vi "log SET errors.vi"(8 "error in (no error)":errorcluster, 11 "Channel in":refnum<class "Channel.lvclass">) -> (0 "error out":errorcluster, 3 "Channel out":refnum<class "Channel.lvclass">)   [LabVIEW 2018, in "Channel.lvclass"]
uses:
  Channel.lvclass
  Channel.lvclass/Channel.ctl
  Sim_Ixon_Ultra/Sim_Ixon_Ultra.lvclass
  C:/Users/Denis/Desktop/S4ACS/S4ACS/Simulated_CCD_Camera/Simulated Camera.lvclass
  Simulated_CCD_Camera/Simulated Camera.lvclass
panel:
  out "SET errors":T1
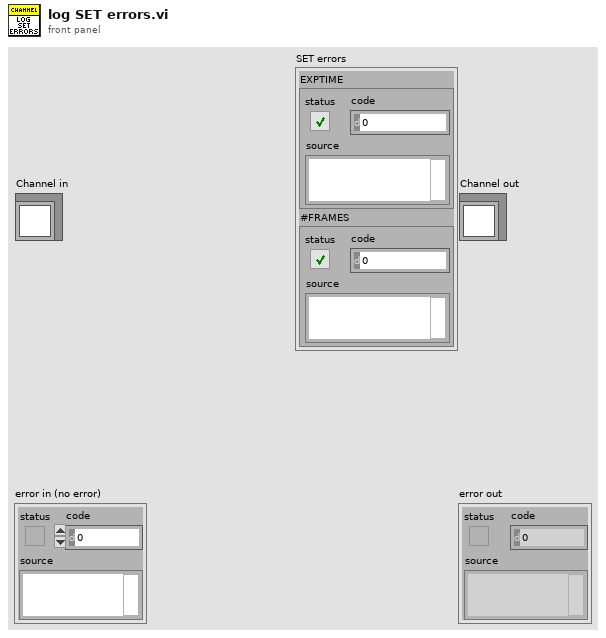
[diagram p1: front panel]
types:
  T1 = cluster{"EXPTIME":errorcluster, "#FRAMES":errorcluster}
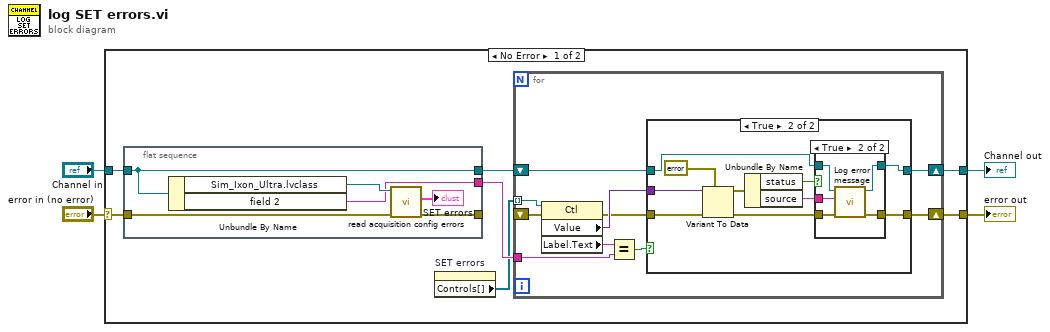
[diagram p0: block diagram]
diagram:
  n1 = case shown="No Error" "error in (no error)" {
    selector: "error in (no error)" -> [w10 w48]
    tunnel: [w7 w48] -> w3
    tunnel: [w8 w47] -> w1
    tunnel: "Channel in" -> [w11 w47]
    frame No Error {
      n2 = flat-sequence {
        tunnel: w11 -> [w17]
        tunnel: w10 -> [w15]
        tunnel: [w17] -> w9
        tunnel: [w14] -> _
        tunnel: [w13] -> w6
        frame #0 {
          n3 = Unbundle By Name(w17) -> ("Sim_Ixon_Ultra.lvclass"=w16:refnum<class "Sim_Ixon_Ultra.lvclass">, "field 2"=w13:string)
          n4 = call "read acquisition config errors.vi"("error in (no error)"=w15, "Simulated Camera in"=w16) -> ("error out"=w14:errorcluster, "SET errors"=→"SET errors":T1)  [unwired: 7 in, 1 out]
        }
      }
      n5 = property on="SET errors" class="Clust (strict)"() -> ("Controls[]"=w5:refnum<vi>[])  [unwired: 2 in, 2 out]
      n6 = for {
        shift-right: [w26] -> w8
        shift-left: w9 -> [w27]
        shift-right: [w25] -> w7
        shift-left: _ -> [w22]
        tunnel: w5 -> [w24] mode=indexing
        tunnel: w6 -> [w19]
        n7 = property class="Ctl"(reference=w24, error in=w22) -> (error out=w21:errorcluster, "Value"=w23:variant, "Label.Text"=w20:string)  [unwired: 1 out]
        n8 = Equal?(x=w20, y=w19) -> (x = y?=w18:bool)
        n9 = case shown="True" w18 {
          tunnel: w27 -> [w29 w39]
          tunnel: [w29 w38] -> w26
          tunnel: [w28 w37] -> w25
          tunnel: w23 -> [_ w36]
          tunnel: w21 -> [w28 w31]
          frame False {
          }
          frame True {
            n10 = Variant To Data(error in=w31, type=errorcluster {"status"=FALSE, "code"=0, "source"=""} ("error constant"), Variant=w36) -> (data=w33:errorcluster, error out=w34:errorcluster)
            n11 = Unbundle By Name(w33) -> ("status"=w30:bool, "source"=w32:string)
            n12 = case shown="True" w30 {
              tunnel: w39 -> [w41 w46]
              tunnel: [w41 w45] -> w38
              tunnel: [w40 w44] -> w37
              tunnel: w34 -> [w40 w43]
              tunnel: w32 -> [_ w42]
              frame False {
              }
              frame True {
                n13 = call "Log error message.vi"("error in (no error)"=w43, "String"=w42, "Channel in"=w46) -> ("error out"=w44:errorcluster, "Channel out"=w45:refnum<class "Channel.lvclass">)  [unwired: 7 in]
              }
            }
          }
        }
      }
    }
    frame Error {
    }
  }
  "error out" <- w3
  "Channel out" <- w1
